vi "Scan Setup.vi"(8 "error in (no error)":errorcluster, 11 "Translation Stage Coarse in":refnum<class "Translation Stage Coarse.lvclass">) -> (0 "error out":errorcluster, 3 "Translation Stage Coarse out":refnum<class "Translation Stage Coarse.lvclass">)   [LabVIEW 2017, in "Translation Stage Coarse.lvclass"]
doc: "Configure the Instrument based on the class member fields. This step comes after the user has closed the \"Scan Setup\" window and before the actual scan -- so instruments are configured with the user's specified settings."
uses:
  Translation Stage Coarse.lvclass
  Translation Stage Coarse.lvclass/Translation Stage Coarse.ctl
  Global/GPIB Numbers.vi
  Scanner/Scanner.lvclass
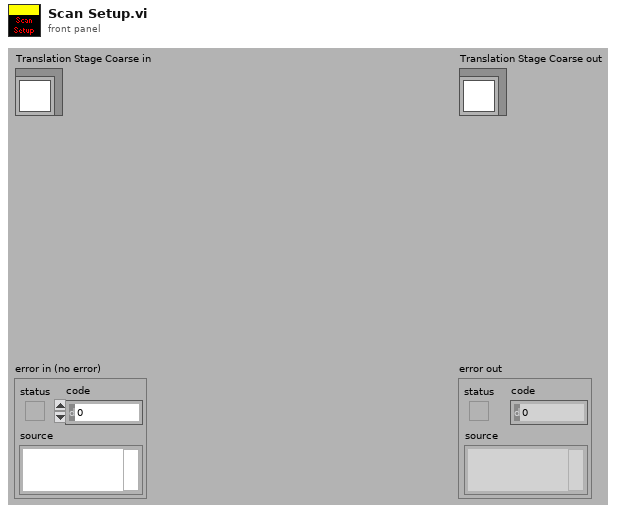
[diagram p1: front panel]
types:
  T1 = typedef "GPIB Type Def.ctl" = cluster{"Name":string, "bus":dbl, "GPIB":dbl, "GPIB as string":string, "byte":i32, "VISA Resource Name":refnum<visa-resource-name>}
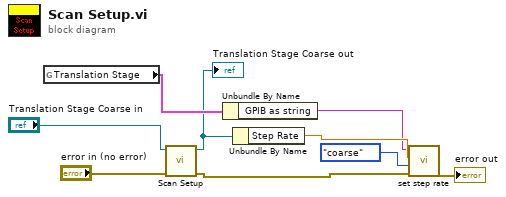
[diagram p0: block diagram]
diagram:
  n1 = global read "GPIB Numbers.vi" "Translation Stage"() -> (w5:T1)
  n2 = call-parent "Scan Setup.vi"("error in (no error)"="error in (no error)", "Scanner in"="Translation Stage Coarse in") -> ("error out"=w2:errorcluster, "Scanner out"=w4:refnum<class "Translation Stage Coarse.lvclass">)  [unwired: 8 in]
  "Translation Stage Coarse out" <- w4
  n3 = Unbundle By Name(w5) -> ("GPIB as string"=w1:string)
  n4 = Unbundle By Name(w4) -> ("Step Rate"=w6:dbl)
  n5 = call "set step rate.vi"("error in"=w2, "axis (def: fine)"=enum16{"fine", "coarse"}."coarse", "step rate"=w6, "GPIB # (in): def. 6"=w1) -> ("error out"=→"error out":errorcluster)  [unwired: 7 out]
